vi "Arduino Move Complete Check.vi"(11 "input string":string) -> (0 "Direction":bool, 1 "Complete?":bool, 2 "position":i32, 3 "m":i32)   [LabVIEW 2024, in "FW Arduino Control.lvclass"]
uses:
  FW Arduino Control.lvclass
  <vilib>/regexp/Match Regular Expression.xnode
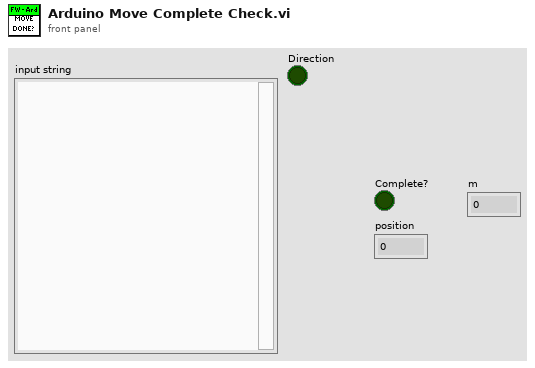
[diagram p1: front panel]
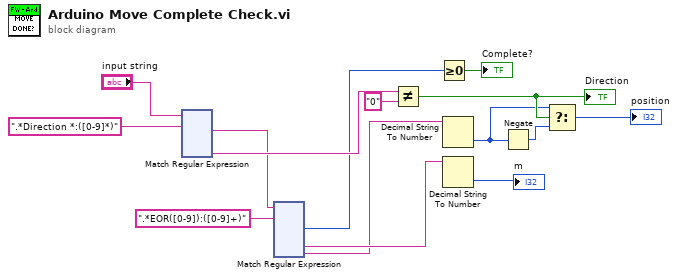
[diagram p0: block diagram]
diagram:
  n1 = xnode "Match Regular Expression"("input string"="input string", "regular expression"=".*Direction *:([0-9]*)") -> ("after match"=w9:string, "submatch 1"=w12:string)  [unwired: 4 in, 4 out]
  n2 = xnode "Match Regular Expression"("input string"=w9, "regular expression"=".*EOR([0-9]):([0-9]+)") -> ("offset past match"=w1:i32, "submatch 1"=w3:string, "submatch 2"=w2:string)  [unwired: 4 in, 4 out]
  n3 = Not Equal?(x=w12, y="0") -> (x != y?=w8:bool)
  "Direction" <- w8
  n4 = Greater Or Equal To 0?(x=w1) -> (x >= 0?=→"Complete?":bool)
  n5 = Decimal String To Number(string=w2) -> (number=w6:i32)  [unwired: 2 in, 1 out]
  n6 = Decimal String To Number(string=w3) -> (number=→"m":i32)  [unwired: 2 in, 1 out]
  n7 = Negate(x=w6) -> (-x=w7:i32)
  n8 = Select(t=w6, s=w8, f=w7) -> (s? t:f=→"position":i32)
